vi "SoftFrontPanel.vi"(8 "error in (no error)":errorcluster, 11 "Scope":refnum<class "Scope Instrument.lvclass">) -> (0 "error out":errorcluster, 3 "Scope out":refnum<class "Scope Instrument.lvclass">)   [LabVIEW 2025, in "Scope.lvlib" / "Scope Instrument.lvclass"]
doc: "Copyright 2017 National Instruments Corporation\n\nLicensed under the Apache License, Version 2.0 (the \"License\"); you may not use this file except in compliance with the License. You may obtain a copy of the License at http://www.apache.org/licenses/LICENSE-2.0\nUnless required by applicable law or agreed to in writing, software distributed under the License is distributed on an \"AS IS\" BASIS, WITHOUT WARRANTIES OR CONDITIONS OF ANY KIND, either express or implied. See the License for the specific language governing permissions and limitations under the License."
uses:
  Scope Instrument.lvclass
  Scope Instrument.lvclass/Scope Instrument.ctl
  Scope configuration/Scope configuration.lvclass
  Users/Public/Documents/Sandia National Labs/TSS Plugin/Abstract Engine.lvlibp/Plugin/Abstract/Instrument configuration/Read Instrument Setting.vi
panel:
  out "Chart Msg":string
  out "Waveform Graph":waveform(dbl)[](graph)
  out "Instrument":string caption="Instrument ::"
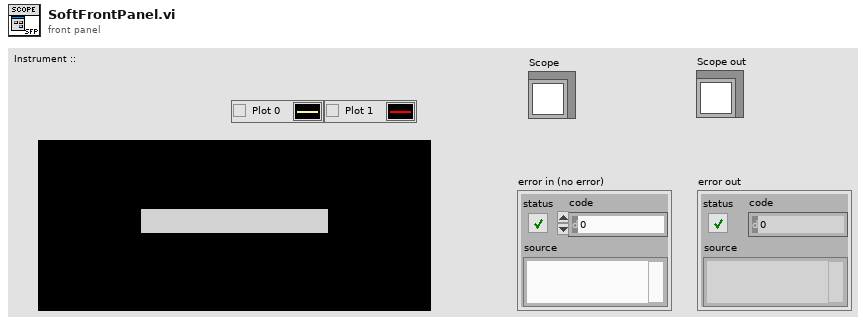
[diagram p1: front panel]
types:
  T1 = enum32{"Invalid", "Default", "Floating", "Floating/Auto-Hide", "Modal"}
  T2 = typedef "Abstract Engine.lvlibp/Instrument configuration.lvclass/Default Instrument.ctl" = cluster{"Type":string, "Address":string, "SW Alias":string, "Description":string, "Enabled":bool}
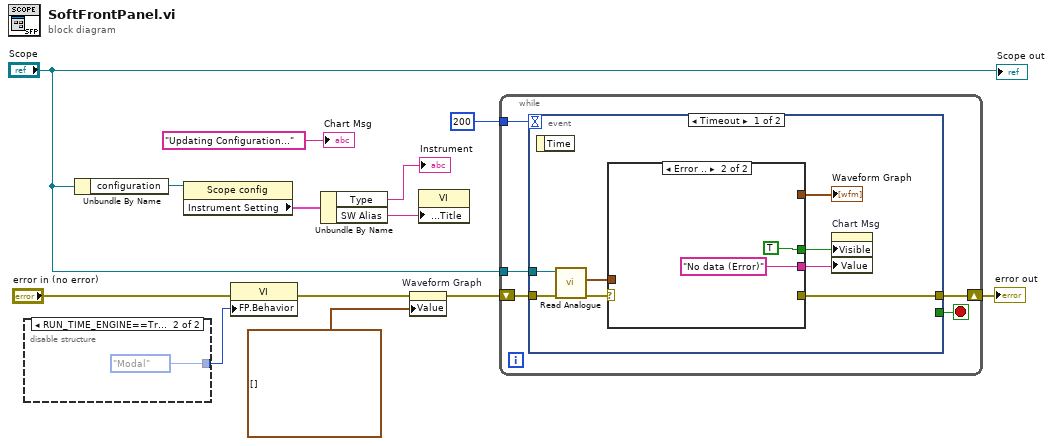
[diagram p0: block diagram]
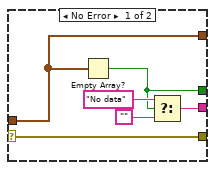
[diagram p2: hidden frame]
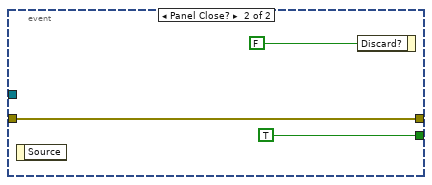
[diagram p3: hidden frame]
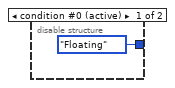
[diagram p4: hidden frame]
diagram:
  n1 = disable-structure shown="RUN_TIME_ENGINE==True" {
    disable-tunnel: [T1."Floating" ("Front Panel Window:Behavior") T1."Modal" ("Front Panel Window:Behavior")] -> w13
    frame condition #0 (active) {
    }
    frame condition #1 {
    }
  }
  n2 = Unbundle By Name("Scope") -> ("configuration"=w7:refnum<class "Scope configuration.lvclass">)
  n3 = property class="Scope config"(reference=w7) -> ("Instrument Setting"=w6:T2)  [unwired: 1 in, 2 out]
  n4 = property class="VI"(error in="error in (no error)", "FP.Behavior"=w13) -> (error out=w11:errorcluster)  [unwired: 1 in, 1 out]
  n5 = Unbundle By Name(w6) -> ("Type"=→"Instrument":string, "SW Alias"=w4:string)
  n6 = property on="Waveform Graph" class="WFGraph (strict)"(error in=w11, "Value"=waveform(dbl)[] [] ("Waveform Graph")) -> (error out=w9:errorcluster)  [unwired: 1 in, 1 out]
  n7 = property class="VI"("Front Panel.Title"=w4) -> ()  [unwired: 2 in, 2 out]
  n8 = while {
    shift-right: [w18] -> w2
    shift-left: w9 -> [w19]
    tunnel: "Scope" -> [w17]
    tunnel: 200 -> [w16]
    stop <- w20 stop-if-true
    n9 = event shown="[0] Timeout" {
      selector: _ -> [_ _]
      dyn-events: _ -> [_ _]
      timeout: w16 -> [_ _]
      tunnel: [_ TRUE] -> w20
      tunnel: [w27 w37] -> w18
      tunnel: w19 -> [w23 w37]
      tunnel: w17 -> [w24 _]
      event Timeout {
        n10 = event-data() -> ()  [unwired: 1 in, 1 out]
        n11 = call-dynamic "Read Analogue.vi"("error in (no error)"=w23, "Analog Input in"=w24) -> ("error out"=w22:errorcluster, "Waveforms"=w21:waveform(dbl)[])  [unwired: 7 in, 1 out]
        n12 = case shown="Error .." w22 {
          selector: w22 -> [w29 _]
          tunnel: [w30 _] -> w28
          tunnel: [w29 _] -> w27
          tunnel: [w32 TRUE ("empty?")] -> w26
          tunnel: [w31 "No data (Error)" ("No data")] -> w25
          tunnel: w21 -> [w30 _]
          frame No Error {
            n13 = Empty Array?(array=w30) -> (empty?=w32:bool)
            n14 = Select(t="No data" ("No data"), s=w32, f="") -> (s? t:f=w31:string)
          }
          frame Error {
          }
        }
        "Waveform Graph" <- w28
        n15 = property on="Chart Msg" class="Str"("Visible"=w26, "Value"=w25) -> ()  [unwired: 2 in, 2 out]
      }
      event Panel Close? {
        n16 = event-data() -> ()  [unwired: 1 in, 1 out]
        n17 = event-data("Discard?"=FALSE) -> ()  [unwired: 1 in, 1 out]
      }
    }
  }
  "error out" <- w2
  "Chart Msg" <- "Updating Configuration..." ("No data")
  "Scope out" <- "Scope"
